vi "Delete StringArray DVR.vi"(8 "error in (no error)":errorcluster, 11 "StringArray DVR in":refnum<data-value>) -> (0 "error out":errorcluster, 3 "StringArray out":refnum<class "StringArray.lvclass">)   [LabVIEW 2013, in "MDSplus.lvlib" / "StringArray.lvclass"]
uses:
  <vilib>/MDSplus/Classes/Data_Class/Array_Class/StringArray_Class/StringArray.lvclass
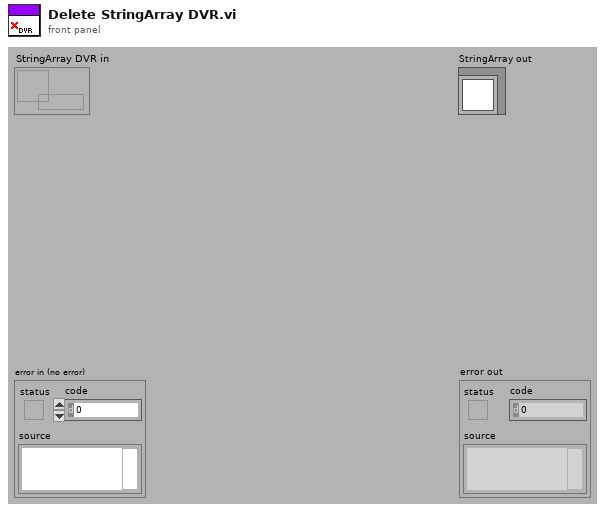
[diagram p1: front panel]
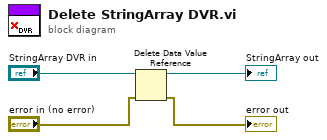
[diagram p0: block diagram]
diagram:
  n1 = Delete Data Value Reference(data value reference="StringArray DVR in", error in="error in (no error)") -> (data value=→"StringArray out":refnum<class "StringArray.lvclass">, error out=→"error out":errorcluster)
